vi "Trav_single_profile.vi"(3 "Simulate/Run":T1, 5 "Traverse line":T2 {"Carrier_2 Q (l/min)" format="%#.2f"; "Row Duration (mins)" format="%#.1f"; "Row No" min=0; "Trace Gas Concentration (%)" min=0.0 format="%#_4f"; "Carrier_1 Q (l/min)" format="%#.4f"; "Start X" format="%#.2f"; "Start Y" format="%#.2f"; "Start Z" format="%#.2f"; "End X" format="%#.2f"; "End Y" format="%#.2f"; "End Z" format="%#.2f"; "Tunnel Speed" format="%#.2f"; "Averaging time (mins)" min=0.0 format="%#.2f"}) -> (0 "Error Messages":string, 1 "Status":T5, 2 "Traverse line Out":T2 {"Carrier_2 Q (l/min)" format="%#.2f"; "Row Duration (mins)" format="%#.1f"; "Row No" min=0; "Trace Gas Concentration (%)" min=0.0 format="%#_4f"; "Carrier_1 Q (l/min)" format="%#.4f"; "Start X" format="%#.2f"; "Start Y" format="%#.2f"; "Start Z" format="%#.2f"; "End X" format="%#.2f"; "End Y" format="%#.2f"; "End Z" format="%#.2f"; "Tunnel Speed" format="%#.2f"; "Averaging time (mins)" min=0.0 format="%#.2f"})   [LabVIEW 2021]
uses:
  Globals/Trav_pos_global.vi
  Globals/Meas_global.vi
  Controls/User_Specific_mode.ctl
  Gen Trav/Multi_Run_Status.ctl
  Controls/Setup.ctl
  Controls/Save_Data.ctl
  Controls/Overhead.ctl
  ADAM Client/Sub VIs/ADAM Controls/Traverse_Level_State.ctl
  Camera Server/Camera enum/Camera resolution.ctl
  Globals/Extra_Commands_Global.vi
  Globals/Preference_global.vi
  Gen Trav/Spacing.ctl
  Gen Trav/Traverse_cluster.ctl
  Controls/Multi_run_mode.ctl
panel:
  in  "pointIDs":string[](array[string])
  out "Point index":i32
  out "Pause message":string
  in  "Pause":bool
  out "Current position":sgl[](array[numeric]) format="%.2f"
  in  "Stop":bool
  in  "Array of Positions":sgl[][](array[numeric]) format="%.2f"
  out "Abcissa copy":string="Y (mm)"
  out "Abcissa":string="Y (mm)"
  in  "ChannelsToPlot":i32[](listbox)=[1]
  out "Started Profile at:":string="16/9/98 12:33"
  out "Currently on point":i32=9
  out "Means":cluster{sgl[], sgl[]}[](graph)
  out "Turbulence%":cluster{sgl[], sgl[]}[](graph)
  # "X           Y          Z"
  # "Start"
  # "End"
  # "X           Y          Z"
  # "Start"
  # "End"
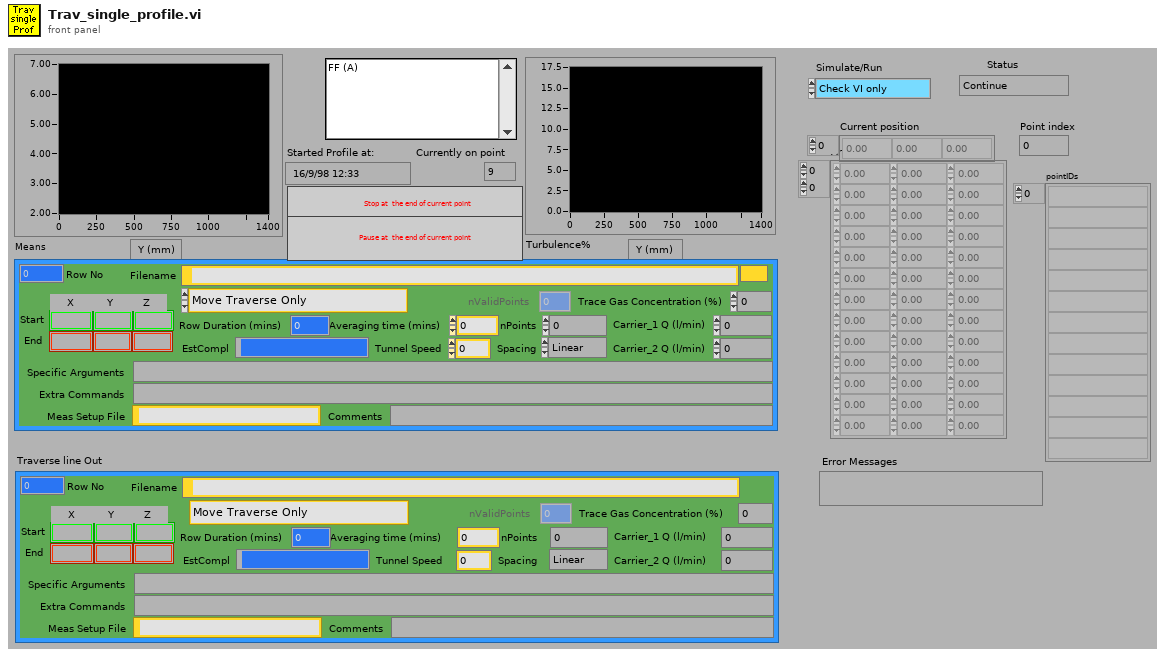
[diagram p1: front panel]
types:
  T1 = typedef "User_Specific_mode.ctl" = enum16{"Check VI only", "Run VI"}
  T2 = typedef "Traverse_cluster.ctl" = cluster{"Start X":sgl, "Start Y":sgl, "Start Z":sgl, "End X":sgl, "End Y":sgl, "End Z":sgl, "nPoints":i32, "Spacing":T3, "Filename":path, "Tunnel Speed":dbl, "Averaging time (mins)":dbl, "Extra Commands":string, "Carrier_1 Q (l/min)":dbl, "Carrier_2 Q (l/min)":dbl, "Trace Gas Concentration (%)":dbl, "Specific Arguments":string, "Comments":string, "Row No":i32, "Row Type Selector":T4, "EstCompl":string, "Row Duration (mins)":dbl, "nValidPoints":i32, "Meas Setup File":string}
  T3 = typedef "Spacing.ctl" = enum16{"Linear", "Log", "Gauss", "Specified", "N/A"}
  T4 = typedef "Multi_run_mode.ctl" = enum16{"Move Traverse Only", "Set Tunnel Speed Only", "Set Source Only", "Set Measurement Conditions", "Single Measurement", "Vertical Profile", "Lateral Profile", "Longitudinal Profile", "Multi-Axis Profile", "Explore Volume", "Auto Calibrate", "Meas Fast FID Bkgnd", "Check Beam Power", "Scanning Valve Measurement", "Run VI Named:", "Set ADAM Ch", "Wait (minutes)", "Send Message", "Synchronize With:", "Fall Back to this Row", "Turn Off Row Repeating", "Traverse 3D Volume", "Blank Row", "Jump to Fall Back Row"}
  T5 = typedef "Multi_Run_Status.ctl" = enum16{"Continue", "Continue with Error", "Jump to Next Point", "Jump to Next Row", "Jump To Fall Back", "Terminate Run"}
  T6 = typedef "Overhead.ctl" = enum16{"Update total times", "Read Current Overhead", "Re Scale totals to 3 hrs", "Initialise totals to 3hr"}
  T7 = typedef "Save_Data.ctl" = enum16{"Save No Data", "Save Data"}
  T8 = typedef "Setup.ctl" = enum16{"Run Program", "Show Setup", "Save Current Setup", "Setup Front Panel"}
  T9 = typedef "Traverse_Level_State.ctl" = enum16{"Running", "Complete"}
  T10 = typedef "GMU Gas Line Name.ctl" = enum16{"GMU1 Source", "GMU2 Source", "GMU2 Calib", "CPP GRC-A", "CPP GRC-B"}
  T11 = typedef "Status_Cluster.ctl" = cluster{"Status":T5, "Error Type":string, "Error Description":string}
  T12 = typedef "Analysis_info_cluster.ctl" = cluster{"Colour":u32, "Inst type":T13, "Inst name":string, "Symbol":string, "Code name":string, "Extra Info":string, "Inst Array":T14, "Extra Titles":string[], "Extra Values":string[], "U":dbl, "u^2":dbl, "u^3":dbl, "u^4":dbl, "Skew_u":dbl, "Kurt_u":dbl, "Sd Error in Mean":dbl, "% u'/U":dbl, "X":dbl, "Y":dbl, "Z":dbl, "Timescale integral Estimate":dbl, "Sd Error in Variance":dbl, "Calib File":path, "Calib Constants":dbl[], "Output Position":bool, "Stats":enum16{"None", "Basic", "Full"}, "Av Sampling Rate":dbl, "Av No of Samples":dbl, "Total Meas Time (s)":dbl, "ADAM Ch Name":string, "Max value":dbl, "Min value":dbl, "Req Sample Rate Hz":dbl, "Sync Delay Time (s)":dbl, "Ch No":i16, "Device":string, "Use Latest Calib":bool, "Port":string, "Metadata Ch Names":string[], "Metadata Ch Values":string[], "Label":string}
  T13 = typedef "Inst_type.ctl" = enum16{"Raw voltage", "Raw with zero offsetting", "Propeller anemometer", "Pressure Transducer", "Pitot-static tube", "Hot wire", "Cross wire 1", "Cross wire 2", "Generic Linear", "Generic Polynomial", "Generic BackPoly", "Fast FID", "Thermocouple", "Cold wire", "Pulsed Wire", "LDA Vel", "LDA Tran time", "LDA Arr time", "Microphone"}
  T14 = typedef "Instrument_Array.ctl" = enum16{"PWA", "LDA", "Analogue"}
  T15 = typedef "Camera resolution.ctl" = u8
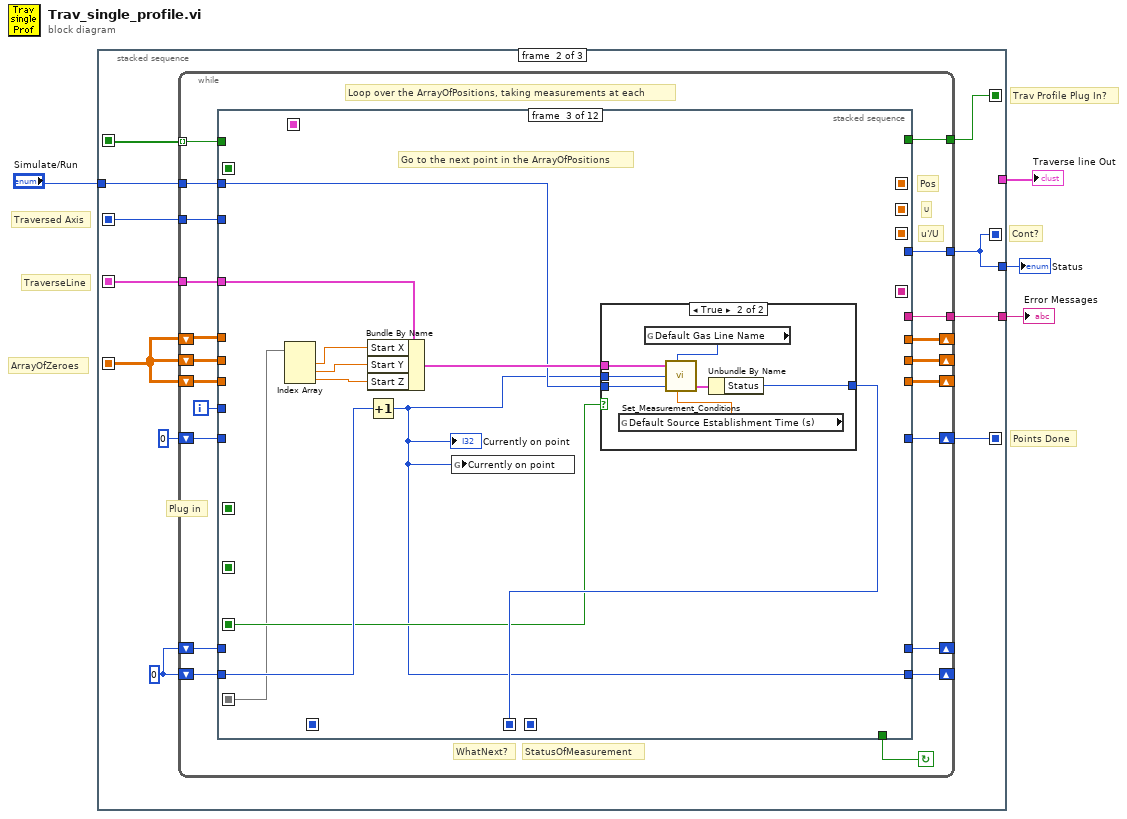
[diagram p0: block diagram]
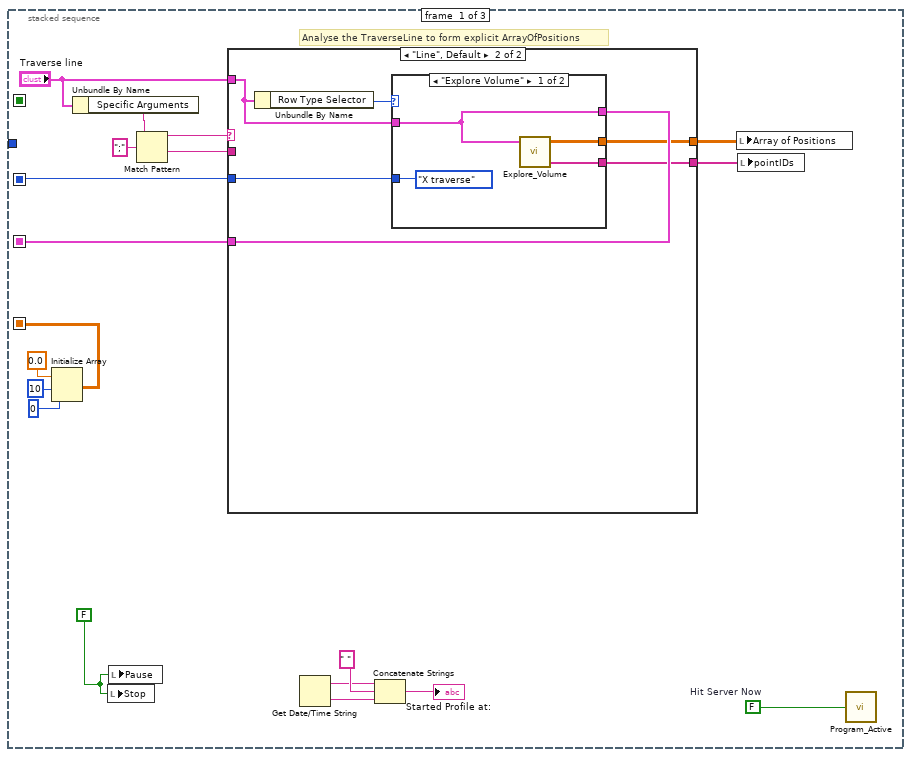
[diagram p2: hidden frame]
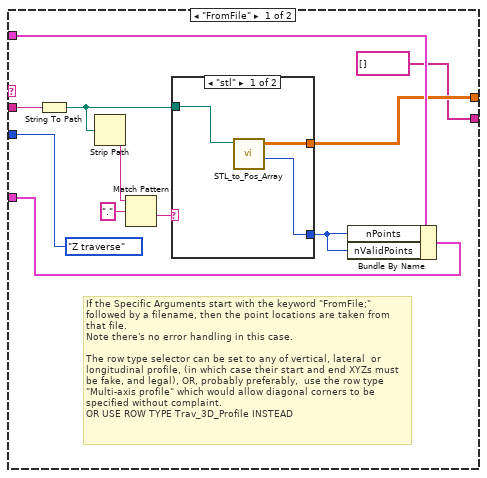
[diagram p3: hidden frame]
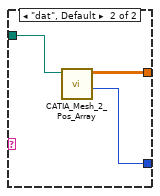
[diagram p4: hidden frame]
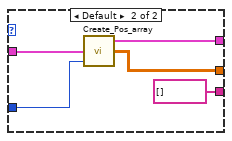
[diagram p5: hidden frame]
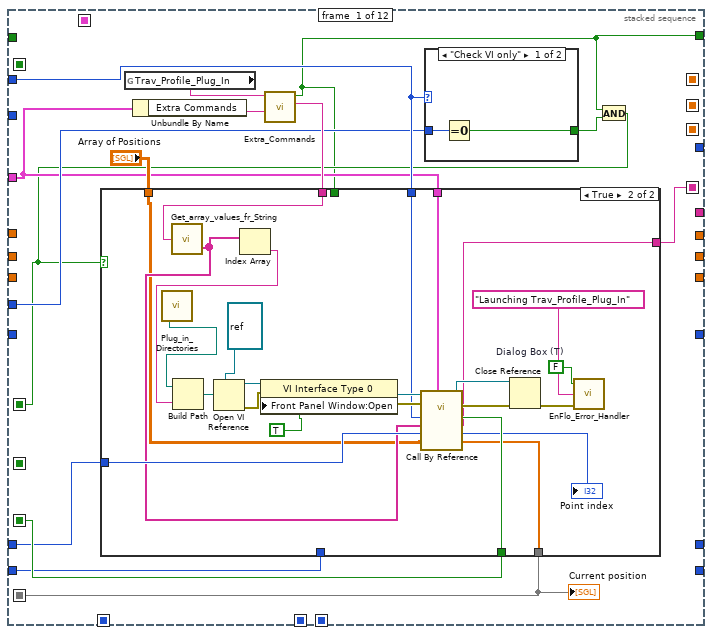
[diagram p6: hidden frame]
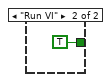
[diagram p7: hidden frame]
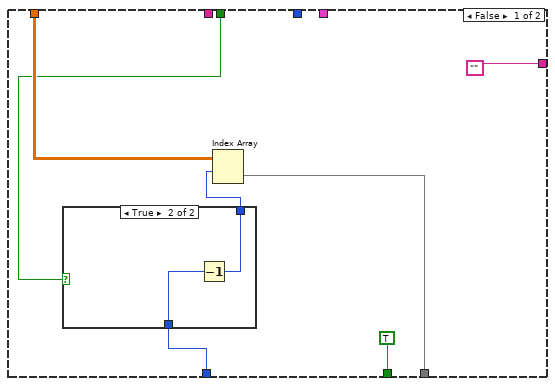
[diagram p8: hidden frame]
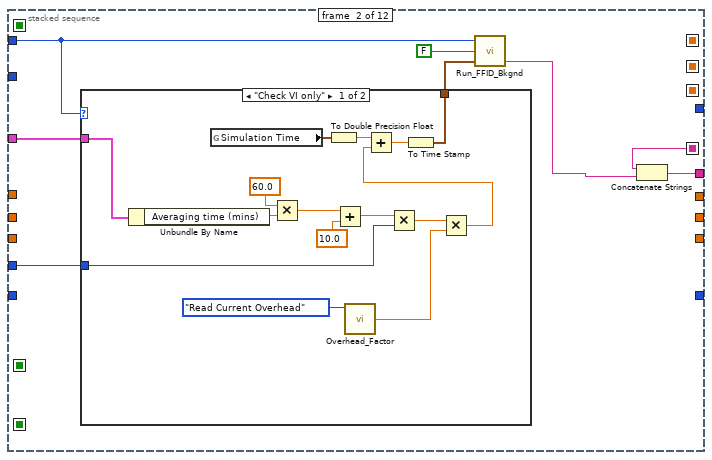
[diagram p10: hidden frame]
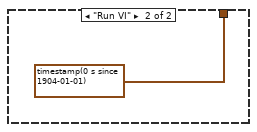
[diagram p11: hidden frame]
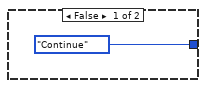
[diagram p12: hidden frame]
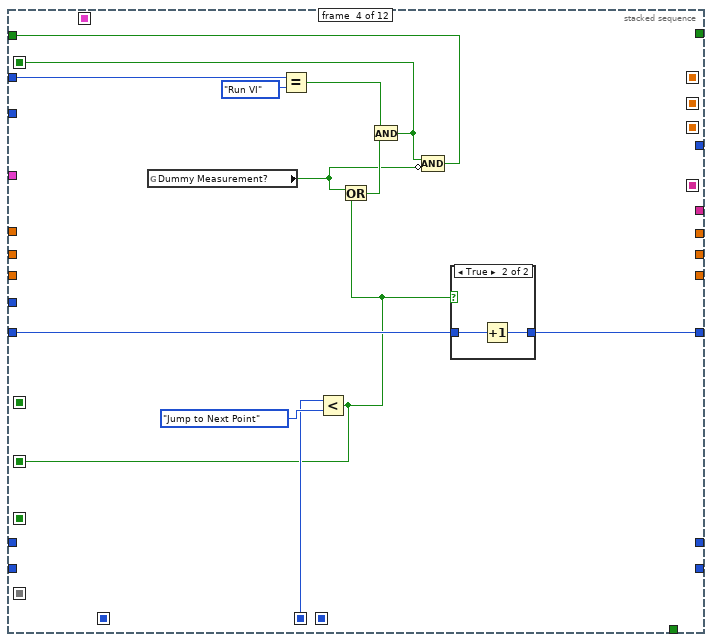
[diagram p13: hidden frame]
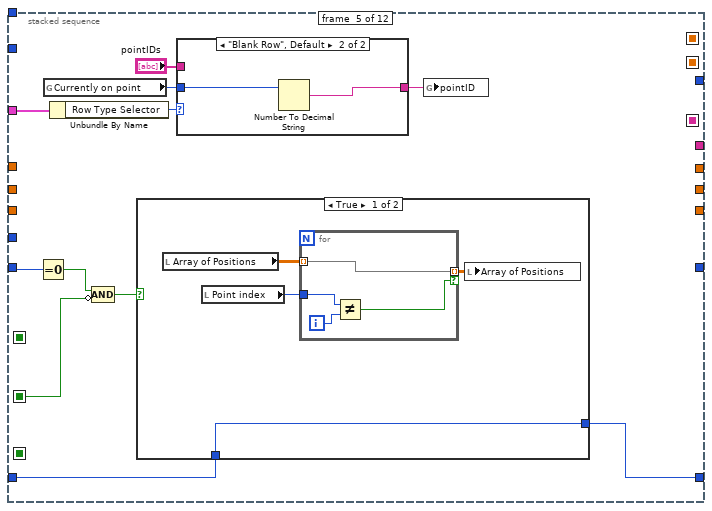
[diagram p15: hidden frame]
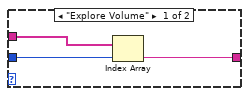
[diagram p16: hidden frame]
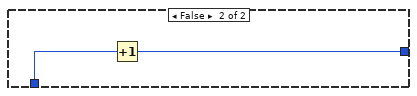
[diagram p17: hidden frame]
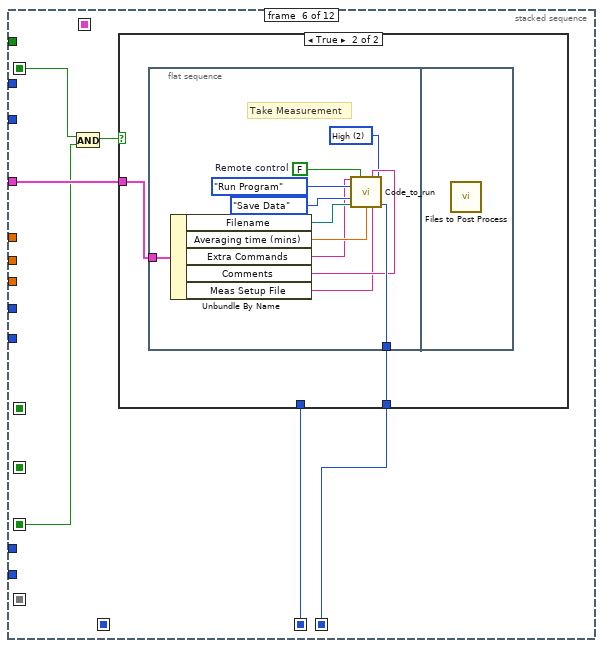
[diagram p18: hidden frame]
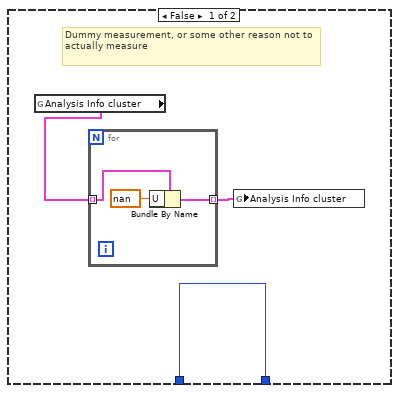
[diagram p19: hidden frame]
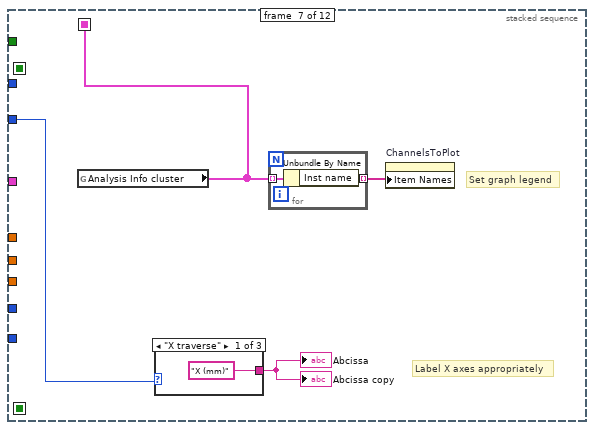
[diagram p20: hidden frame]
diagram:
  # "Trav Profile Plug In?"
  # "ArrayOfZeroes"
  # "TraverseLine"
  # "Traversed Axis"
  # "Points Done"
  # "Cont?"
  n1 = stacked-sequence {
    seq-local: [w16 _ _] -> [_ w65 _]
    seq-local: [w15 _ _] -> [_ w66 _]
    seq-local: [_ w64 _] -> [_ _ _]
    seq-local: [_ w62 _] -> [_ _ _]
    seq-local: [_ w60 _] -> [_ _ w381]
    seq-local: [w12 _ _] -> [_ w59 w380]
    seq-local: [_ w57 _] -> [_ _ w379]
    tunnel: [_ w64 _] -> w2
    tunnel: [_ _ w392] -> w4
    tunnel: "Simulate/Run" -> [_ w63 w391]
    tunnel: [_ w58 _] -> w1
    frame #0 {
      w13 = FALSE ("stop")
      w14 = FALSE  # Hit Server Now
      # "Analyse the TraverseLine to form explicit ArrayOfPositions"
      n2 = Initialize Array(sgl 0.0, 10, 0) -> (w16:sgl[][])
      n3 = Unbundle By Name("Traverse line") -> ("Specific Arguments"=w9:string)
      n4 = local write "Stop"(w13) -> ()
      n5 = local write "Pause"(w13) -> ()
      n6 = Match Pattern(string=w9, regular expression=";") -> (before substring=w7:string, after substring=w6:string)  [unwired: 1 in, 2 out]
      n7 = case shown="\"Line\", Default" w7 {
        tunnel: [enum16{"X traverse", "Y traverse", "Z traverse"}."Z traverse" ("Axis Traversed") w46] -> w15
        tunnel: "Traverse line" -> [w28 w43]
        tunnel: [w27 w45] -> w12
        tunnel: [w25 w44] -> w11
        tunnel: w6 -> [w29 _]
        tunnel: [string[] [] ("pointIDs") w41] -> w5
        frame "FromFile" {
          # "If the Specific Arguments start with the keyword \"FromFile;\" followed by a filename, then the point locations are taken from that file.\nNote there's no error handling in this case.\n\nThe row type selector can be set to any of vertical, lateral  or longitudinal profile, (in which case their start and end XYZs must be fake, and legal), OR, probably preferably,  use the row type \"Multi-axis profile\" which would allow diagonal corners to be specified without complaint.\nOR USE ROW TYPE Trav_3D_Profile INSTEAD"
          n8 = String To Path(string=w29) -> (path=w31:path)
          n9 = Strip Path(path=w31) -> (name=w33:string)  [unwired: 1 out]
          n10 = Match Pattern(string=w33, regular expression=".") -> (after substring=w34:string)  [unwired: 1 in, 3 out]
          n11 = case shown="\"stl\"" w34 {
            tunnel: [w36 w40] -> w25
            tunnel: [w35 w39] -> w30
            tunnel: w31 -> [w37 w38]
            frame "stl" {
              n12 = call "STL_to_Pos_Array.vi"("STL file"=w37) -> ("Number of Points"=w35:i32, "Array of Positions"=w36:dbl[][])  [unwired: 9 in]
            }
            frame "dat", Default {
              n13 = call "CATIA_Mesh_2_Pos_Array.vi"("Catia Mesh File"=w38) -> ("Number of Points"=w39:i32, "Array of Positions"=w40:dbl[][])  [unwired: 9 in]
            }
          }
          n14 = Bundle By Name(cluster=w28, "nPoints"=w30, "nValidPoints"=w30) -> (w27:T2)
        }
        frame "Line", Default {
          n15 = Unbundle By Name(w43) -> ("Row Type Selector"=w42:T4)
          n16 = case shown="\"Explore Volume\"" w42 {
            tunnel: [enum16{"X traverse", "Y traverse", "Z traverse"}."X traverse" ("Axis Traversed") w55] -> w46
            tunnel: w43 -> [w50 w54]
            tunnel: [w50 w53] -> w45
            tunnel: [w49 w52] -> w44
            tunnel: [w47 string[] [] ("pointIDs")] -> w41
            frame "Explore Volume" {
              n17 = call "Explore_Volume.vi"("Traverse line In"=w50) -> ("pointIDs"=w47:string[], "Position Array"=w49:sgl[][])  [unwired: 3 in]
            }
            frame Default {
              n18 = call "Create_Pos_array.vi"("Traverse line"=w54) -> ("Traverse line Out"=w53:T2, "Array of Positions"=w52:sgl[][], "Axis Traversed"=w55:enum16{"X traverse", "Y traverse", "Z traverse"})  [unwired: 5 in, 1 out]
            }
          }
        }
      }
      n19 = Get Date/Time String() -> (date string=w22:string, time string=w21:string)  [unwired: 3 out]
      n20 = Concatenate Strings(w22, " ", w21) -> (→"Started Profile at:":string)
      n21 = local write "Array of Positions"(w11) -> ()
      n22 = local write "pointIDs"(w5) -> ()
      n23 = call "Program_Active.vi"("Hit Server Now"=w14) -> ()
    }
    frame #1 {
      w56 = 0
      # "Plug in"
      n24 = while {
        shift-left: 0 -> [w74]
        shift-right: [w73] -> w60
        tunnel: [w75] -> w62 mode=indexing
        tunnel: w59 -> [w76]
        tunnel: w63 -> [w77]
        tunnel: [w78] -> w64
        shift-left: w65 -> [w81]
        shift-right: [w80] -> _
        tunnel: w66 -> [w82]
        shift-left: w65 -> [w84]
        shift-right: [w83] -> _
        shift-left: w65 -> [w86]
        shift-right: [w85] -> _
        tunnel: [w72] -> w58
        shift-right: [w70] -> _
        shift-left: w56 -> [w71]
        tunnel: [w69] -> w57
        shift-right: [w67] -> _
        shift-left: w56 -> [w68]
        i -> [w87]
        stop <- w79 continue-if-true
        # "StatusOfMeasurement"
        # "WhatNext?"
        # "Loop over the ArrayOfPositions, taking measurements at each"
        # "Pos"
        # "U"
        # "u'/U"
        n25 = stacked-sequence {
          seq-local: [_ _ _ _ _ _ w249 _ _ _ _ _] -> [_ _ _ _ _ _ _ w263 _ w299 _ _]
          seq-local: [_ _ _ _ _ _ _ w259 _ _ _ _] -> [_ _ _ _ _ _ _ _ w289 _ _ _]
          seq-local: [_ _ _ _ _ _ _ w261 _ _ _ _] -> [_ _ _ _ _ _ _ _ w288 _ _ _]
          seq-local: [_ _ _ _ _ _ _ w262 _ _ _ _] -> [_ _ _ _ _ _ _ _ w287 _ _ _]
          seq-local: [_ _ _ _ _ _ _ _ "ChannelsToPlot" _ _ _] -> [_ _ _ _ _ _ _ _ _ w305 _ _]
          seq-local: [_ _ _ _ _ w229 _ _ _ _ _ _] -> [_ _ _ _ _ _ _ _ _ _ _ w365]
          seq-local: [_ _ w171 _ _ _ _ _ _ _ _ _] -> [_ _ _ w184 _ w228 _ _ _ _ _ _]
          seq-local: [_ _ _ w187 _ _ _ _ _ _ _ _] -> [_ _ _ _ _ w226 _ _ _ _ _ _]
          seq-local: [w99 _ _ _ _ _ _ _ _ _ _ _] -> [_ _ w167 _ _ w225 _ _ _ _ _ w361]
          seq-local: [w98 _ _ _ _ _ _ _ _ _ _ _] -> [_ w144 _ _ _ _ _ _ _ _ _ _]
          seq-local: [w93 _ _ _ _ _ _ _ _ _ _ _] -> [_ _ w166 _ _ _ _ _ _ _ _ _]
          seq-local: [w90 _ _ _ _ _ _ _ _ _ _ _] -> [_ _ _ _ _ _ _ _ _ _ _ w358]
          seq-local: [_ _ _ w183 _ _ _ _ _ _ _ _] -> [_ _ _ _ w206 _ _ _ _ _ _ _]
          tunnel: w87 -> [w96 w145 _ _ _ _ _ _ _ _ _ _]
          tunnel: w86 -> [_ _ _ _ _ _ _ w265 _ _ _ _]
          tunnel: [_ _ _ _ _ _ _ w261 _ _ _ _] -> w85
          tunnel: w84 -> [_ _ _ _ _ _ _ w264 _ _ _ _]
          tunnel: [_ _ _ _ _ _ _ w262 _ _ _ _] -> w83
          tunnel: w82 -> [_ _ _ _ _ _ w251 w258 _ _ _ _]
          tunnel: w81 -> [_ _ _ _ _ _ _ w260 _ _ _ _]
          tunnel: [_ _ _ _ _ _ _ w259 _ _ _ _] -> w80
          tunnel: [_ _ _ _ _ _ _ _ _ _ _ w360] -> w79
          tunnel: w76 -> [w92 w146 w164 _ w202 w227 _ _ _ _ _ _]
          tunnel: [_ _ _ _ _ _ _ _ _ _ _ w359] -> w78
          tunnel: w77 -> [w97 w147 w172 w194 _ _ _ _ _ _ _ _]
          tunnel: [_ _ _ w188 _ _ _ _ _ _ _ _] -> w75
          tunnel: w74 -> [_ _ _ w191 w208 _ _ _ _ _ _ _]
          tunnel: [_ _ _ w190 _ _ _ _ _ _ _ _] -> w73
          tunnel: [_ w142 _ _ _ _ _ _ _ _ _ _] -> w72
          tunnel: w71 -> [w91 _ w168 _ _ _ _ _ _ _ _ w357]
          tunnel: [_ _ w165 _ _ _ _ _ _ _ _ _] -> w70
          tunnel: [w89 _ _ _ _ _ _ _ _ _ _ _] -> w69
          tunnel: w68 -> [w88 _ _ _ w204 _ _ _ _ _ _ _]
          tunnel: [_ _ _ _ w203 _ _ _ _ _ _ _] -> w67
          frame #0 {
            n26 = global read "Extra_Commands_Global.vi" "Trav_Profile_Plug_In"() -> (w102:string)
            n27 = Unbundle By Name(w92) -> ("Extra Commands"=w101:string)
            n28 = call "Extra_Commands.vi"("String to Search"=w101, "Command"=w102) -> ("String Value"=w100:string, "Command Found"=w89:bool)  [unwired: 1 in, 3 out]
            n29 = case shown="\"Check VI only\"" w97 {
              tunnel: w96 -> [w104 _]
              tunnel: [w103 TRUE] -> w95
              frame "Check VI only" {
                n30 = Equal To 0?(x=w104) -> (x = 0?=w103:bool)
              }
              frame "Run VI" {
              }
            }
            n31 = And(x=w89, y=w95) -> (x .and. y?=w90:bool)
            n32 = case shown="True" w90 {
              tunnel: w100 -> [_ w138]
              tunnel: w88 -> [_ w124]
              tunnel: [TRUE ("Stop") w123] -> w99
              tunnel: w97 -> [_ w122]
              tunnel: ["" w120] -> w98
              tunnel: w91 -> [w107 _]
              tunnel: "Array of Positions" -> [w110 w119]
              tunnel: [w109 w118] -> w93
              tunnel: w92 -> [_ w117]
              tunnel: w89 -> [w108 _]
              frame False {
                n33 = case shown="True" w108 {
                  tunnel: w107 -> [w113 w115]
                  tunnel: [w113 w114] -> w106
                  frame False {
                  }
                  frame True {
                    n34 = Decrement(x=w115) -> (x-1=w114:i32)
                  }
                }
                n35 = Index Array(array=w110, index (row)=w106) -> (element=w109:sgl[])  [unwired: 1 in]
              }
              frame True {
                w134 = FALSE  # Dialog Box (T)
                n36 = call "Plug_in_Directories.vi"() -> ("Trav_Profile_Plug_Ins"=w139:path)  [unwired: 2 in, 4 out]
                n37 = call "Get_array_values_fr_String.vi"("String Value"=w138) -> ("String array"=w121:string[])  [unwired: 1 out]
                n38 = Index Array(array=w121) -> (element=w137:string)  [unwired: 1 in]
                n39 = Build Path(base path=w139, name or relative path=w137) -> (appended path=w129:path)
                n40 = Open VI Reference(type specifier VI Refnum (for type only)=refnum<vi> refnum ("Plug in"), vi path=w129) -> (vi reference=w132:refnum<vi>, error out=w131:errorcluster)  [unwired: 2 in, 2 out]
                n41 = property class="VI Interface Type 0"(reference=w132, error in=w131, "Front Panel Window:Open"=TRUE ("Wait until done")) -> (reference out=w128:refnum<vi>, error out=w127:errorcluster)
                n42 = call-by-ref "?"(reference=w128, error in=w127, "Traverse line"=w117, "Array of Positions"=w119, "Loop i"=w124, "Arguments"=w121, "Simulate/Run"=w122) -> (reference out=w126:refnum<vi>, error out=w125:errorcluster, "Next Position"=w118:sgl[], "Point index"=→"Point index":i32, "Error String"=w120:string, "Continue"=w123:bool)
                n43 = Close Reference(reference=w126, error in (no error)=w125) -> (error out=w135:errorcluster)
                n44 = call "EnFlo_Error_Handler.vi"("error in (no error)"=w135, "Error Type"="Launching Trav_Profile_Plug_In", "Dialog Box (F)"=w134) -> ()  [unwired: 3 out]
              }
            }
            "Current position" <- w93
          }
          frame #1 {
            n45 = case shown="\"Check VI only\"" w147 {
              tunnel: w146 -> [w162 _]
              tunnel: w145 -> [w148 _]
              tunnel: [w151 timestamp(0 s since 1904-01-01)] -> w141
              frame "Check VI only" {
                n46 = Unbundle By Name(w162) -> ("Averaging time (mins)"=w159:dbl)
                n47 = global read "Trav_pos_global.vi" "Simulation Time"() -> (w153:timestamp)
                n48 = Multiply(x=60.0, y=w159) -> (x*y=w158:dbl)
                n49 = To Double Precision Float(number=w153) -> (double precision float=w154:dbl)
                n50 = Add(x=w158, y=10.0 ("Scalable Time (Sec)")) -> (x+y=w157:dbl)
                n51 = call "Overhead_Factor.vi"("Mode"=Overhead."Read Current Overhead") -> ("Current Overhead Factor"=w149:dbl)  [unwired: 3 in]
                n52 = Multiply(x=w157, y=w148) -> (x*y=w150:dbl)
                n53 = Multiply(x=w150, y=w149) -> (x*y=w155:dbl)
                n54 = Add(x=w154, y=w155) -> (x+y=w152:dbl)
                n55 = To Time Stamp(1:w152) -> (0:w151:timestamp)
              }
              frame "Run VI" {
              }
            }
            n56 = call "Run_FFID_Bkgnd.vi"("Simulated Time"=w141, "Run Now?"=FALSE, "Simulate/Run"=w147) -> ("Error Messages"=w143:string)  [unwired: 2 out]
            n57 = Concatenate Strings(w144, w143) -> (w142:string)
          }
          frame #2 {
            # "Go to the next point in the ArrayOfPositions"
            n58 = Index Array(array=w166) -> (element #1=w174:sgl, element #2=w170:sgl, element #3=w169:sgl)  [unwired: 3 in]
            n59 = Bundle By Name(cluster=w164, "Start X"=w174, "Start Y"=w170, "Start Z"=w169) -> (w173:T2)
            n60 = Increment(x=w168) -> (x+1=w165:i32)
            "Currently on point" <- w165
            n61 = global write "Trav_pos_global.vi" "Currently on point"(w165) -> ()
            n62 = case shown="True" w167 {
              tunnel: w173 -> [_ w182]
              tunnel: w172 -> [_ w181]
              tunnel: [Multi_Run_Status."Continue" ("Status") w179] -> w171
              tunnel: w165 -> [_ w178]
              frame False {
              }
              frame True {
                n63 = global read "Preference_global.vi" "Default Source Establishment Time (s)"() -> (w176:dbl)
                n64 = global read "Trav_pos_global.vi" "Default Gas Line Name"() -> (w177:T10)
                n65 = call "Set_Measurement_Conditions.vi"("Traverse line"=w182, "Gas Line Name"=w177, "Currently on Point"=w178, "Simulate/Run"=w181, "Source Establishment Time (s)"=w176) -> ("Status Cluster"=w180:T11)  [unwired: 2 in]
                n66 = Unbundle By Name(w180) -> ("Status"=w179:T5)
              }
            }
          }
          frame #3 {
            n67 = global read "Trav_pos_global.vi" "Dummy Measurement?"() -> (w186:bool)
            n68 = Equal?(x=w194, y=User_Specific_mode."Run VI" ("Simulate/Run")) -> (x = y?=w192:bool)
            n69 = Less?(x=w184, y=Multi_Run_Status."Jump to Next Point" ("Status")) -> (x < y?=w183:bool)
            n70 = Or(x=w186, y=w183) -> (x .or. y?=w189:bool)
            n71 = And(x=w192, y=w189) -> (x .and. y?=w187:bool)
            n72 = Compound Arithmetic op=AND(w187, invert w186) -> (w188:bool)
            n73 = case shown="True" w183 {
              tunnel: w191 -> [w195 w197]
              tunnel: [w195 w196] -> w190
              frame False {
              }
              frame True {
                n74 = Increment(x=w197) -> (x+1=w196:i32)
              }
            }
          }
          frame #4 {
            n75 = Equal To 0?(x=w208) -> (x = 0?=w207:bool)
            n76 = global read "Trav_pos_global.vi" "Currently on point"() -> (w200:i32)
            n77 = Unbundle By Name(w202) -> ("Row Type Selector"=w201:T4)
            n78 = Compound Arithmetic op=AND(w207, invert w206) -> (w205:bool)
            n79 = case shown="True" w205 {
              tunnel: w204 -> [w214 w223]
              tunnel: [w214 w222] -> w203
              frame True {
                n80 = local read "Array of Positions"() -> (w216:sgl[][])
                n81 = local read "Point index"() -> (w215:i32)
                n82 = for {
                  tunnel: [w221] -> w217 mode=indexing if=w218
                  tunnel: w216 -> [w221] mode=indexing
                  tunnel: w215 -> [w219]
                  i -> [w220]
                  n83 = Not Equal?(x=w219, y=w220) -> (x != y?=w218:bool)
                }
                n84 = local write "Array of Positions"(w217) -> ()
              }
              frame False {
                n85 = Increment(x=w223) -> (x+1=w222:i32)
              }
            }
            n86 = case shown="\"Blank Row\", Default" w201 {
              tunnel: w200 -> [w211 w213]
              tunnel: "pointIDs" -> [w210 _]
              tunnel: [w209 w212] -> w198
              frame "Explore Volume" {
                n87 = Index Array(array=w210, index=w211) -> (element=w209:string)
              }
              frame "Blank Row", Default {
                n88 = Number To Decimal String(number=w213) -> (decimal integer string=w212:string)  [unwired: 1 in]
              }
            }
            n89 = global write "Trav_pos_global.vi" "pointID"(w198) -> ()
          }
          frame #5 {
            n90 = And(x=w226, y=w225) -> (x .and. y?=w224:bool)
            n91 = case shown="True" w224 {
              tunnel: [w232 w237] -> w229
              tunnel: w228 -> [w232 _]
              tunnel: w227 -> [_ w236]
              frame False {
                # "Dummy measurement, or some other reason not to actually measure"
                n92 = global read "Meas_global.vi" "Analysis Info cluster"() -> (w231:T12[])
                n93 = for {
                  tunnel: w231 -> [w235] mode=indexing
                  tunnel: [w233] -> w230 mode=indexing
                  n94 = Bundle By Name(cluster=w235, "U"=nan) -> (w233:T12)
                }
                n95 = global write "Meas_global.vi" "Analysis Info cluster"(w230) -> ()
              }
              frame True {
                n96 = flat-sequence {
                  tunnel: [w248] -> w237
                  tunnel: w236 -> [w242]
                  frame #0 {
                    w239 = T15 2 items=["Low", "Med.", "High", "Max."] ("Camera Resolution")
                    w247 = FALSE  # Remote control
                    # "Take Measurement"
                    n97 = Unbundle By Name(w242) -> ("Filename"=w245:path, "Averaging time (mins)"=w246:dbl, "Extra Commands"=w241:string, "Comments"=w240:string, "Meas Setup File"=w238:string)
                    n98 = call "Code_to_run.vi"("Extra command String"=w241, "Current Row Comments"=w240, "Camera Resolution"=w239, "setup"=Setup."Run Program", "Remote control"=w247, "File"=Save_Data."Save Data", "Results Filename"=w245, "Averaging time (min)"=w246, "Setup filename"=w238) -> ("Status"=w248:T5)  [unwired: 3 in, 3 out]
                  }
                  frame #1 {
                    n99 = call "Files to Post Process.vi"() -> ()  [unwired: 12 in]
                  }
                }
              }
            }
          }
          frame #6 {
            # "Label X axes appropriately"
            # "Set graph legend"
            n100 = global read "Meas_global.vi" "Analysis Info cluster"() -> (w249:T12[])
            n101 = case shown="\"X traverse\"" w251 {
              tunnel: ["X (mm)" "Y (mm)" "Z (mm)"] -> w250
              frame "X traverse" {
              }
              frame "Y traverse" {
              }
              frame "Z traverse" {
              }
            }
            "Abcissa" <- w250
            "Abcissa copy" <- w250
            n102 = for {
              tunnel: w249 -> [w257] mode=indexing
              tunnel: [w256] -> w252 mode=indexing
              n103 = Unbundle By Name(w257) -> ("Inst name"=w256:string)
            }
            n104 = property on="ChannelsToPlot" class="LstBox (strict)"("Item Names"=w252) -> ()  [unwired: 2 in, 2 out]
          }
          frame #7 {
            # "Accumulate plot data"
            n105 = for {
              tunnel: w265 -> [w283] mode=indexing
              tunnel: [w281] -> w261 mode=indexing
              tunnel: w264 -> [w280] mode=indexing
              tunnel: [w278] -> w262 mode=indexing
              tunnel: w263 -> [w277] mode=indexing
              tunnel: w260 -> [w276] mode=indexing
              tunnel: [w275] -> w259 mode=indexing
              tunnel: w258 -> [w270]
              n106 = Unbundle By Name(w277) -> ("X"=w274:dbl, "Y"=w273:dbl, "Z"=w272:dbl, "U"=w282:dbl, "% u'/U"=w279:dbl)
              n107 = To Single Precision Float(number=w279) -> (single precision float=w268:sgl)
              n108 = To Single Precision Float(number=w282) -> (single precision float=w269:sgl)
              n109 = Build Array(w274, w273, w272) -> (w271:dbl[])
              n110 = Index Array(array=w271, index=w270) -> (element=w267:dbl)
              n111 = To Single Precision Float(number=w267) -> (single precision float=w266:sgl)
              n112 = Build Array (concatenate)(w276, w266) -> (w275:sgl[])
              n113 = Build Array (concatenate)(w283, w269) -> (w281:sgl[])
              n114 = Build Array (concatenate)(w280, w268) -> (w278:sgl[])
            }
          }
          frame #8 {
            n115 = for {
              tunnel: "ChannelsToPlot" -> [w290] mode=indexing
              tunnel: w289 -> [w298]
              tunnel: w288 -> [w297]
              tunnel: w287 -> [w296]
              tunnel: [w292] -> w286 mode=indexing
              tunnel: [w291] -> w285 mode=indexing
              n116 = Index Array(array=w298, index (row)=w290) -> (element=w294:sgl[])  [unwired: 1 in]
              n117 = Index Array(array=w297, index (row)=w290) -> (element=w295:sgl[])  [unwired: 1 in]
              n118 = Index Array(array=w296, index (row)=w290) -> (element=w293:sgl[])  [unwired: 1 in]
              n119 = Bundle(w294, w295) -> (w291:cluster{sgl[], sgl[]})  [unwired: 1 out]
              n120 = Bundle(w294, w293) -> (w292:cluster{sgl[], sgl[]})  [unwired: 1 out]
            }
            "Means" <- w285
            "Turbulence%" <- w286
          }
          frame #9 {
            # "add some empty plot names"
            n121 = for {
              tunnel: w305 -> [w309] mode=indexing
              tunnel: w299 -> [w307]
              tunnel: [w306] -> w302 mode=indexing
              n122 = Index Array(array=w307, index=w309) -> (element=w308:T12)
              n123 = Unbundle By Name(w308) -> ("Inst name"=w306:string)
            }
            n124 = Initialize Array("", 5) -> (w301:string[])
            n125 = Build Array (concatenate)(w302, w301) -> (w300:string[])
            n126 = for {
              tunnel: w300 -> [w310] mode=indexing
              i -> [w312]
              n127 = To Unsigned Long Integer(number=w312) -> (unsigned 32bit integer=w311:u32)
              n128 = property on="Means" class="XYGraph (strict)"("Active Plot"=w311, "Plot.Plot Name"=w310) -> ()  [unwired: 2 in, 2 out]
              n129 = property on="u'/U" class="XYGraph (strict)"("Active Plot"=w311, "Plot.Plot Name"=w310) -> ()  [unwired: 2 in, 2 out]
            }
          }
          frame #10 {
            w313 = -1
            # "Check in with server, and pause if requested"
            n130 = while {
              shift-left: w313 -> [w314]
              shift-right: [w315] -> _
              shift-left: w313 -> [w318]
              shift-right: [w319] -> _
              stop <- w316 continue-if-true
              n131 = Increment(x=w318) -> (x+1=w317:i32)
              n132 = case shown="0, Default" w318 {
                tunnel: [w324 w327 w331 w341 w344 w348 0] -> w319
                tunnel: w317 -> [w324 w327 w333 w341 w344 w348 _]
                tunnel: [TRUE ("Pause") "Pause" TRUE ("Pause") TRUE ("Pause") TRUE ("Pause") TRUE ("Pause") TRUE ("Pause")] -> w316
                tunnel: [w323 w326 w329 w338 w342 w346 w351] -> w315
                tunnel: w314 -> [w323 w326 w329 w338 w342 w346 w352]
                frame -1 {
                  # "Report to server"
                  n133 = call "Program_Active_Client.vi"("Mode"=enum16{"Program Active", "Traverse Level State"}."Program Active", "Time till next contact (Sec)"=12000.0, "Traverse level State"=Traverse_Level_State."Running") -> ()  [unwired: 3 out]
                }
                frame 0, Default {
                  # "If user wants to pause..."
                }
                frame 1 {
                  n134 = Quotient & Remainder(x=w329, y=15) -> (x-y*floor(x/y)=w335:i32)  [unwired: 1 out]
                  n135 = global write "Trav_pos_global.vi" "Paused During Row?"(TRUE ("Paused During Row?")) -> ()
                  n136 = Equal To 0?(x=w335) -> (x = 0?=w334:bool)
                  n137 = Increment(x=w333) -> (x+1=w332:i32)
                  n138 = Select(t=w333, s=w334, f=w332) -> (s? t:f=w331:i32)
                }
                frame 2 {
                  # "Bring to front occasionally to remind user we're paused"
                  n139 = Current VI's Path() -> (path=w339:path)
                  n140 = call "Bring_to_front.vi"("path"=w339) -> ()
                }
                frame 3 {
                  # "Write to big indcator, and then flash on and off"
                  "Pause message" <- "Multi Run Program Paused!!!!" ("Pause message")
                }
                frame 4 {
                  n141 = property on="Pause message" class="Str"("Visible"=TRUE) -> ()  [unwired: 2 in, 2 out]
                  n142 = Wait Until Next ms Multiple(millisecond multiple=u32 1500) -> ()  [unwired: 1 out]
                }
                frame 5 {
                  n143 = Increment(x=w352) -> (x+1=w351:i32)
                  n144 = property on="Pause message" class="Str"("Visible"=FALSE) -> ()  [unwired: 2 in, 2 out]
                  n145 = Wait Until Next ms Multiple(millisecond multiple=u32 1500) -> ()  [unwired: 1 out]
                }
              }
            }
          }
          frame #11 {
            n146 = case shown="False" w358 {
              tunnel: [w369 TRUE] -> w363
              tunnel: w357 -> [w368 _]
              frame False {
                n147 = local read "Array of Positions"() -> (w370:sgl[][])
                n148 = Array Size(array=w370) -> (size(s)=w373:i32[])
                n149 = Index Array(array=w373, index=0 ("Index")) -> (element=w371:i32)
                n150 = Increment(x=w368) -> (x+1=w367:i32)
                n151 = Less?(x=w367, y=w371) -> (x < y?=w369:bool)
              }
              frame True {
              }
            }
            n152 = case shown="\"Continue with Error\"" w365 {
              tunnel: [TRUE TRUE TRUE FALSE] -> w362
              frame "Continue" {
              }
              frame "Continue with Error" {
              }
              frame "Jump to Next Point" {
              }
              frame "Jump to Next Row", Default {
              }
            }
            n153 = Compound Arithmetic op=AND(invert "Stop", w363, w362, w361) -> (w360:bool)
            n154 = Select(t=Multi_Run_Status."Terminate Run" ("Status"), s="Stop", f=w365) -> (s? t:f=w359:T5)
          }
        }
      }
    }
    frame #2 {
      n155 = local read "Array of Positions"() -> (w384:sgl[][])
      n156 = Array Size(array=w384) -> (size(s)=w386:i32[])
      n157 = Index Array(array=w386, index=0 ("Index")) -> (element=w383:i32)
      n158 = Not Equal?(x=w383, y=w381) -> (x != y?=w389:bool)
      n159 = Equal?(x=User_Specific_mode."Run VI" ("Simulate/Run"), y=w391) -> (x = y?=w388:bool)
      n160 = Bundle By Name(cluster=w380, "nValidPoints"=w381) -> (w382:T2)
      n161 = Compound Arithmetic op=AND(invert w379, w388, w389) -> (w387:bool)
      n162 = case shown="True" w387 {
        tunnel: w382 -> [w393 w400]
        tunnel: [w393 w407] -> w392
        tunnel: w381 -> [_ w406]
        frame False {
        }
        frame True {
          w401 = " !!Program added comments"
          n163 = Unbundle By Name(w400) -> ("Row No"=w399:i32)
          n164 = Equal To 0?(x=w406) -> (x = 0?=w397:bool)
          n165 = Format Into String(format string="!!(Row %d of Cmd file ", w399) -> (resulting string=w396:string)  [unwired: 2 in, 1 out]
          n166 = case shown="False" w397 {
            tunnel: ["Partially Skipped)" "Skipped)"] -> w395
            frame False {
            }
            frame True {
            }
          }
          n167 = Unbundle By Name(w400) -> ("Comments"=w402:string)
          n168 = Match Pattern(string=w402, regular expression=w401) -> (match substring=w404:string)  [unwired: 4 out]
          n169 = Concatenate Strings(w396, w395) -> (w394:string)
          n170 = Empty String/Path?(string/path=w404) -> (empty?=w403:bool)
          n171 = case shown="False" w403 {
            tunnel: [w412 w416] -> w405
            tunnel: w394 -> [w411 w415]
            tunnel: w401 -> [_ w414]
            tunnel: w402 -> [w410 w413]
            frame False {
              n172 = Concatenate Strings(w410, w411) -> (w412:string)
            }
            frame True {
              n173 = Concatenate Strings(w413, w414, w415) -> (w416:string)
            }
          }
          n174 = Bundle By Name(cluster=w400, "Comments"=w405) -> (w407:T2)
        }
      }
    }
  }
  "Status" <- w2
  "Traverse line Out" <- w4
  "Error Messages" <- w1
